vi "Quickie label 2x1_5 GX430T.vi"() -> ()   [LabVIEW 2013]
panel:
  out "ZPL":string
  in  "Copies":u32=1
  in  "print 2":bool
  in  "print":bool
  in  "Font size 5":u32=14
  in  "Font size 4":u32=14
  in  "Font size 3":u32=14
  in  "Font size 2":u32=14
  in  "line 5":string
  in  "line 4":string
  in  "line 3":string
  in  "line 2":string
  in  "Font size 1":u32=14
  in  "line 1":string
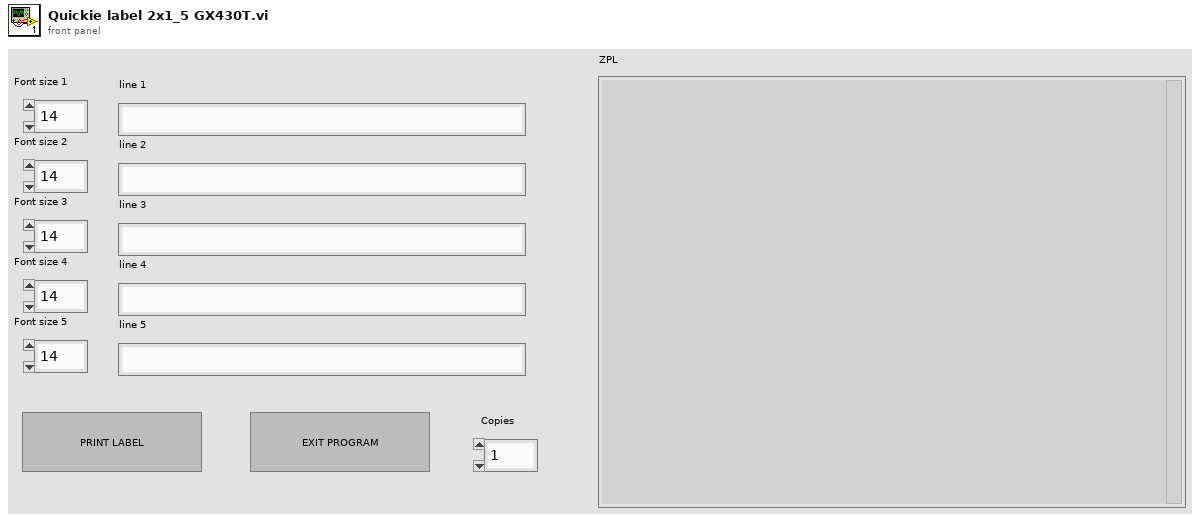
[diagram p1: front panel]
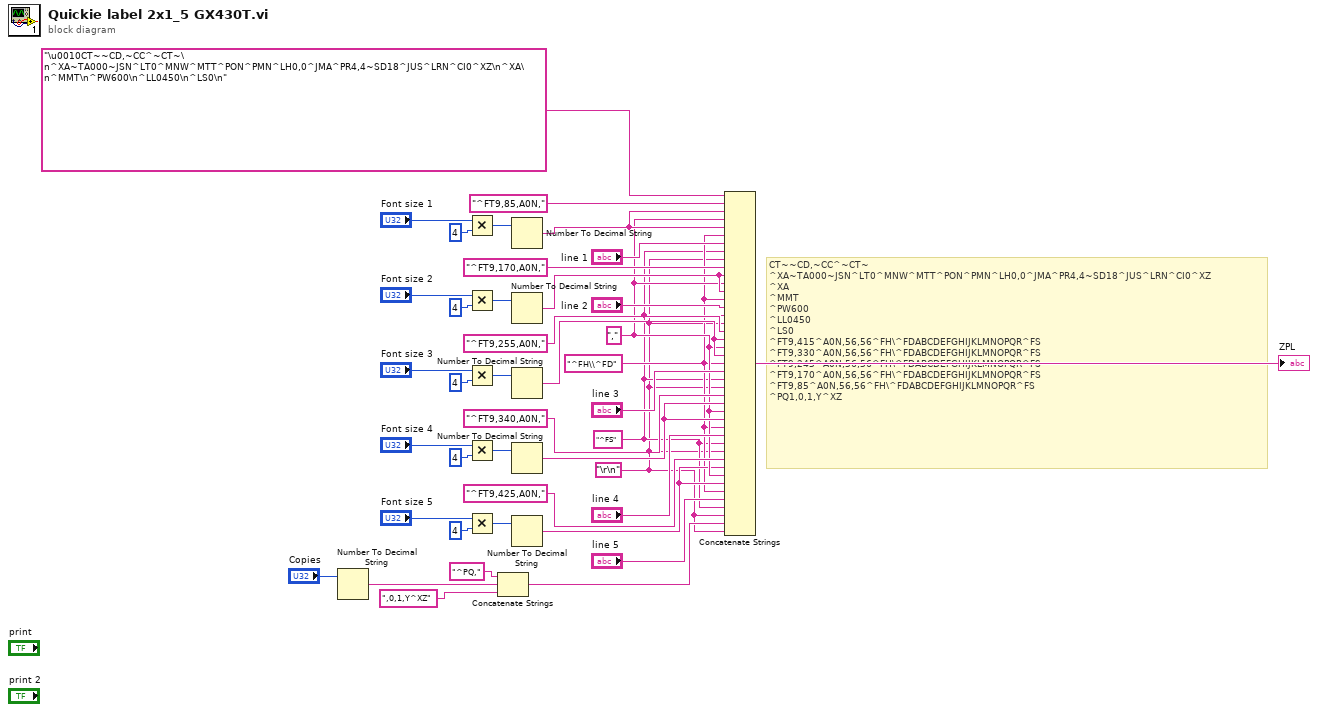
[diagram p0: block diagram]
diagram:
  w1 = "\r\n"
  w4 = "^FS" ("string")
  w6 = "^FH\\^FD" ("string")
  w8 = "," ("string")
  # "CT~~CD,~CC^~CT~\n^XA~TA000~JSN^LT0^MNW^MTT^PON^PMN^LH0,0^JMA^PR4,4~SD18^JUS^LRN^CI0^XZ\n^XA\n^MMT\n^PW600\n^LL0450\n^LS0\n^FT9,415^A0N,56,56^FH\\^FDABCDEFGHIJKLMNOPQR^FS\n^FT9,330^A0N,56,56^FH\\^FDABCDEFGHIJKLMNOPQR^FS\n^FT9,245^A0N,56,56^FH\\^FDABCDEFGHIJKLMNOPQR^FS\n^FT9,170^A0N,56,56^FH\\^FDABCDEFGHIJKLMNOPQR^FS\n^FT9,85^A0N,56,56^FH\\^FDABCDEFGHIJKLMNOPQR^FS\n^PQ1,0,1,Y^XZ"
  n1 = Number To Decimal String(number="Copies") -> (decimal integer string=w39:string)  [unwired: 1 in]
  n2 = Multiply(x="Font size 1", y=u32 4) -> (x*y=w33:u32)
  n3 = Multiply(x="Font size 2", y=u32 4) -> (x*y=w30:u32)
  n4 = Multiply(x="Font size 3", y=u32 4) -> (x*y=w27:u32)
  n5 = Multiply(x="Font size 4", y=u32 4) -> (x*y=w26:u32)
  n6 = Multiply(x="Font size 5", y=u32 4) -> (x*y=w23:u32)
  n7 = Concatenate Strings("^PQ," ("string"), w39, ",0,1,Y^XZ" ("string")) -> (w2:string)
  n8 = Number To Decimal String(number=w33) -> (decimal integer string=w32:string)  [unwired: 1 in]
  n9 = Number To Decimal String(number=w30) -> (decimal integer string=w17:string)  [unwired: 1 in]
  n10 = Number To Decimal String(number=w27) -> (decimal integer string=w14:string)  [unwired: 1 in]
  n11 = Number To Decimal String(number=w26) -> (decimal integer string=w11:string)  [unwired: 1 in]
  n12 = Number To Decimal String(number=w23) -> (decimal integer string=w7:string)  [unwired: 1 in]
  n13 = Concatenate Strings("\u0010CT~~CD,~CC^~CT~\n^XA~TA000~JSN^LT0^MNW^MTT^PON^PMN^LH0,0^JMA^PR4,4~SD18^JUS^LRN^CI0^XZ\n^XA\n^MMT\n^PW600\n^LL0450\n^LS0\n", "^FT9,85,A0N,", w32, w8, w32, w6, "line 1", w4, w1, "^FT9,170,A0N,", w17, w8, w17, w6, "line 2", w4, w1, "^FT9,255,A0N,", w14, w8, w14, w6, "line 3", w4, w1, "^FT9,340,A0N,", w11, w8, w11, w6, "line 4", w4, w1, "^FT9,425,A0N,", w7, w8, w7, w6, "line 5", w4, w1, w2, w1) -> (→"ZPL":string)
